vi "Start Channels if Not Active.vi"(8 "error in":errorcluster, 10 "channels":u8[](array[numeric]), 11 "module handle in":u8) -> (0 "error out":errorcluster, 3 "module handle out":u8)   [LabVIEW 2020, in "AIM ARINC 429 Hardware API.lvlib"]
uses:
  AIM ARINC 429 Hardware API.lvlib
  <instrlib>/AIM GmbH/ARINC-429/subvi/Error Converter (ErrCode or Status).vi
  <instrlib>/AIM GmbH/ARINC-429/subvi/Get Library Path.vi
  <instrlib>/AIM GmbH/ARINC-429/VIs/Library/Api429Lib Error Desc Get.vi
  <instrlib>/AIM GmbH/ARINC-429/subvi/Get Error Number Offset.vi
  <vilib>/Utility/error.llb/Error Cluster From Error Code.vi
  <instrlib>/AIM GmbH/ARINC-429/AIM429LV.lvlib
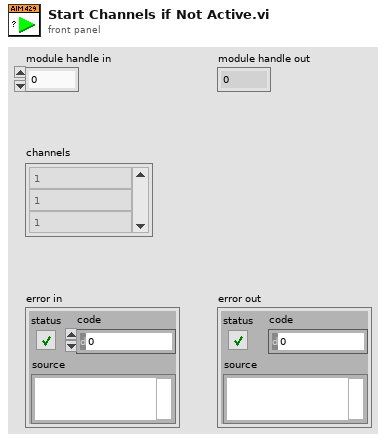
[diagram p1: front panel]
types:
  T1 = typedef "AIM429LV.lvlib/Channel Info Raw.ctl" = cluster{"config_flags":u32, "capability_flags":u32, "speed":u32, "active":u8}
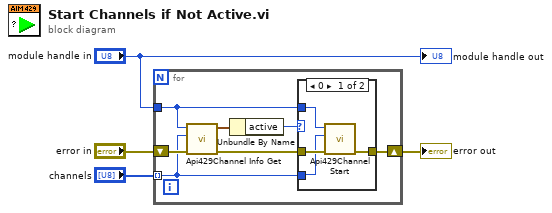
[diagram p0: block diagram]
diagram:
  n1 = for {
    shift-right: [w6] -> w1
    shift-left: "error in" -> [w10]
    tunnel: "module handle in" -> [w5]
    tunnel: "channels" -> [w7] mode=indexing
    n2 = call <instrlib>:"Api429Channel Info Get.vi"("error in (no error)"=w10, "channel_id"=w7, "board_handle"=w5) -> ("error out"=w8:errorcluster, "pxInfo out"=w11:T1)  [unwired: 7 in]
    n3 = Unbundle By Name(w11) -> ("active"=w9:u8)
    n4 = case shown="0" w9 {
      tunnel: w8 -> [w14 w16]
      tunnel: w7 -> [w12 _]
      tunnel: [w13 w16] -> w6
      tunnel: w5 -> [w15 _]
      frame 0 {
        n5 = call <instrlib>:"Api429Channel Start.vi"("error in (no error)"=w14, "channel_id"=w12, "board_handle"=w15) -> ("error out"=w13:errorcluster)  [unwired: 8 in]
      }
      frame Default {
      }
    }
  }
  "error out" <- w1
  "module handle out" <- "module handle in"
